vi "value_to_color.vi"(0 "Tab Control":enum32{"Page 1", "Page 2"}(tab)) -> ()   [LabVIEW 2019]
panel:
  in  "Rang":u16(ring) items=["10^-2", "10^-1", "10^0", "10^1", "10^2", "10^3", "10^4", "10^5", "10^6", "10^7", "10^8", "10^9"]
  in  "4B":bool
  in  "1B":bool
  in  "?":bool
  in  "Decimal value":dbl min=0.0 max=999.0 step=1.0
  in  "Thermal coefficient":u16(ring) items=["200"=200, "100"=100, "50"=50, "15"=15, "25"=25, "10"=10, "5"=5, "1"=1]
  in  "Precision":u16(ring) items=["20 %", "10 %", "5 %", "1 %", "2 %", "0,5 %", "0,25 %", "0,10 %", "0,05 %"]
  in  "6B":bool
  in  "5B":bool
  out "?":string
  in  "ok":bool
  out "L1":bool
  out "L4":bool
  out "L5":bool
  out "L6":bool
  out "L2":bool
  out "L3":bool
  # "Value                                                 Color"
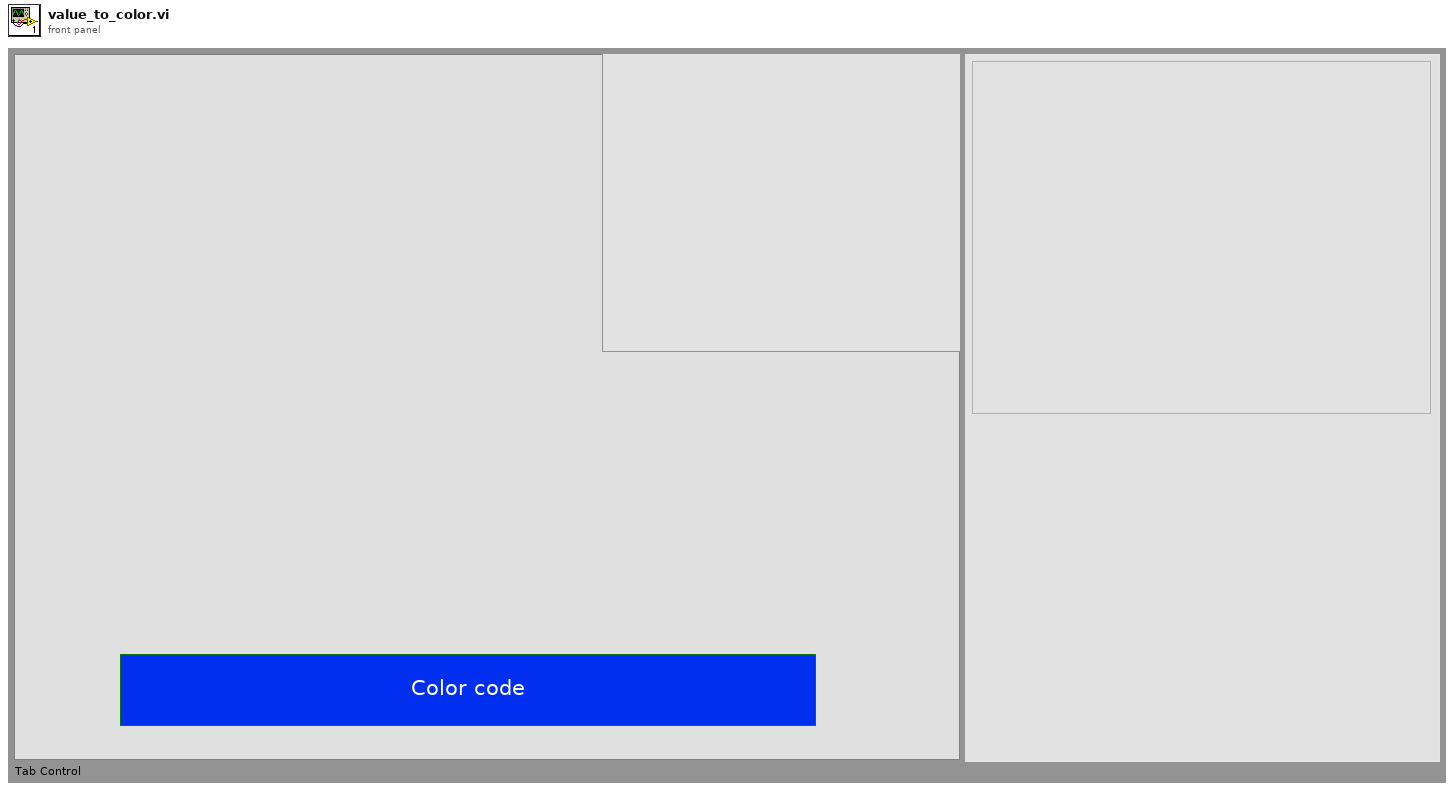
[diagram p1: front panel]
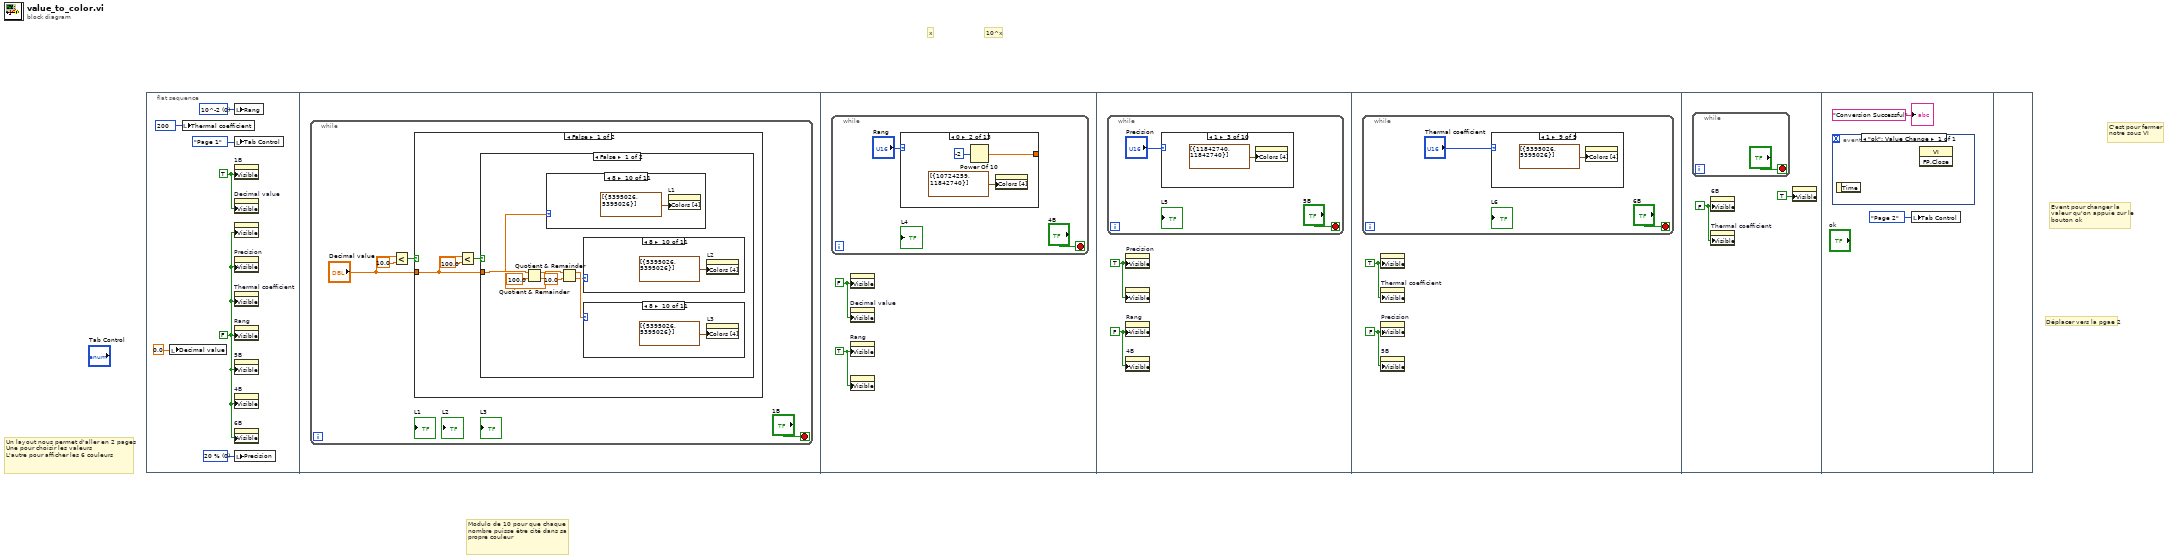
[diagram p0: block diagram]
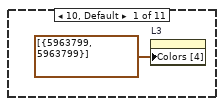
[diagram p2: hidden frame]
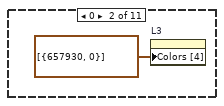
[diagram p3: hidden frame]
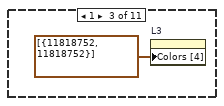
[diagram p4: hidden frame]
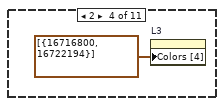
[diagram p5: hidden frame]
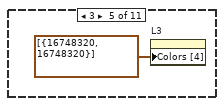
[diagram p6: hidden frame]
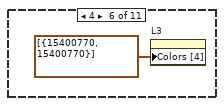
[diagram p7: hidden frame]
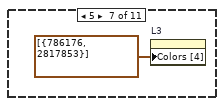
[diagram p8: hidden frame]
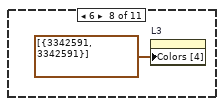
[diagram p9: hidden frame]
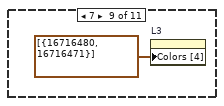
[diagram p10: hidden frame]
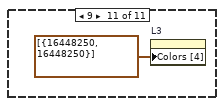
[diagram p11: hidden frame]
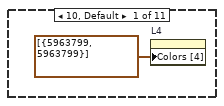
[diagram p12: hidden frame]
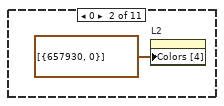
[diagram p13: hidden frame]
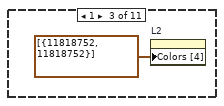
[diagram p14: hidden frame]
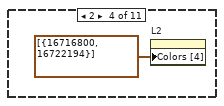
[diagram p15: hidden frame]
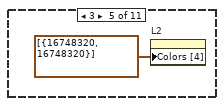
[diagram p16: hidden frame]
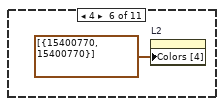
[diagram p17: hidden frame]
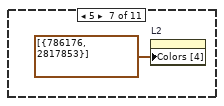
[diagram p18: hidden frame]
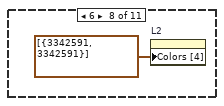
[diagram p19: hidden frame]
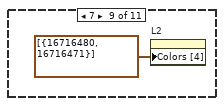
[diagram p20: hidden frame]
diagram:
  # "Déplacer vers la pgae 2"
  # "C'est pour fermer notre sous VI"
  # "Event pour changer la valeur qu'on appuie sur le bouton ok"
  # "x"
  # "10^x"
  # "Modulo de 10 pour que chaque nombre puisse être cité dans sa propre couleur"
  # "Un layout nous permet d'aller en 2 pages\nUne pour choisir les valeurs\nL'autre pour afficher les 6 couleurs"
  n1 = flat-sequence {
    frame #0 {
      w1 = u16 0 items=["20 %", "10 %", "5 %", "1 %", "2 %", "0,5 %", "0,25 %", "0,10 %", "0,05 %"] ("Precision")
      w2 = u16 0 items=["10^-2", "10^-1", "10^0", "10^1", "10^2", "10^3", "10^4", "10^5", "10^6", "10^7", "10^8", "10^9"] ("Rang")
      w3 = u16 200 items=["200"=200, "100"=100, "50"=50, "15"=15, "25"=25, "10"=10, "5"=5, "1"=1] ("Thermal coefficient")
      w7 = TRUE
      w5 = FALSE
      n2 = local write "Decimal value"(0.0 ("Decimal value")) -> ()
      n3 = local write "Thermal coefficient"(w3) -> ()
      n4 = local write "Rang"(w2) -> ()
      n5 = local write "Tab Control"(enum32{"Page 1", "Page 2"}."Page 1" ("Tab Control")) -> ()
      n6 = property on="1B" class="Bool"("Visible"=w7) -> ()  [unwired: 2 in, 2 out]
      n7 = property on="Decimal value" class="DigNum (strict)"("Visible"=w7) -> ()  [unwired: 2 in, 2 out]
      n8 = property class="Bool"("Visible"=w5) -> ()  [unwired: 2 in, 2 out]
      n9 = property on="Precision" class="Ring (strict)"("Visible"=w5) -> ()  [unwired: 2 in, 2 out]
      n10 = property on="Thermal coefficient" class="Ring (strict)"("Visible"=w5) -> ()  [unwired: 2 in, 2 out]
      n11 = property on="Rang" class="Ring (strict)"("Visible"=w5) -> ()  [unwired: 2 in, 2 out]
      n12 = property on="5B" class="Bool"("Visible"=w5) -> ()  [unwired: 2 in, 2 out]
      n13 = property on="4B" class="Bool"("Visible"=w5) -> ()  [unwired: 2 in, 2 out]
      n14 = property on="6B" class="Bool"("Visible"=w5) -> ()  [unwired: 2 in, 2 out]
      n15 = local write "Precision"(w1) -> ()
    }
    frame #1 {
      n16 = while {
        stop <- "1B" stop-if-true
        n17 = Less?(x="Decimal value", y=10.0) -> (x < y?=w8:bool)
        n18 = case shown="False" w8 {
          tunnel: "Decimal value" -> [w12 w84]
          frame False {
            n19 = Less?(x=w12, y=100.0) -> (x < y?=w13:bool)
            n20 = case shown="False" w13 {
              tunnel: w12 -> [w20 w58]
              frame False {
                n21 = Quotient & Remainder(x=w20, y=100.0) -> (x-y*floor(x/y)=w18:dbl, floor(x/y)=w19:dbl)
                n22 = case shown="8" w19 {
                  frame 10, Default {
                    n23 = property on="L1" class="Bool (strict)"("Colors [4]"=cluster{u32, u32}[] [{5963799, 5963799}]) -> ()  [unwired: 2 in, 2 out]
                  }
                  frame 0 {
                    n24 = property on="L1" class="Bool (strict)"("Colors [4]"=cluster{u32, u32}[] [{657930, 0}]) -> ()  [unwired: 2 in, 2 out]
                  }
                  frame 1 {
                    n25 = property on="L1" class="Bool (strict)"("Colors [4]"=cluster{u32, u32}[] [{11818752, 11818752}]) -> ()  [unwired: 2 in, 2 out]
                  }
                  frame 2 {
                    n26 = property on="L1" class="Bool (strict)"("Colors [4]"=cluster{u32, u32}[] [{16716800, 16722194}]) -> ()  [unwired: 2 in, 2 out]
                  }
                  frame 3 {
                    n27 = property on="L1" class="Bool (strict)"("Colors [4]"=cluster{u32, u32}[] [{16748320, 16748320}]) -> ()  [unwired: 2 in, 2 out]
                  }
                  frame 4 {
                    n28 = property on="L1" class="Bool (strict)"("Colors [4]"=cluster{u32, u32}[] [{15400770, 15400770}]) -> ()  [unwired: 2 in, 2 out]
                  }
                  frame 5 {
                    n29 = property on="L1" class="Bool (strict)"("Colors [4]"=cluster{u32, u32}[] [{786176, 2817853}]) -> ()  [unwired: 2 in, 2 out]
                  }
                  frame 6 {
                    n30 = property on="L1" class="Bool (strict)"("Colors [4]"=cluster{u32, u32}[] [{3342591, 3342591}]) -> ()  [unwired: 2 in, 2 out]
                  }
                  frame 7 {
                    n31 = property on="L1" class="Bool (strict)"("Colors [4]"=cluster{u32, u32}[] [{16716480, 16716471}]) -> ()  [unwired: 2 in, 2 out]
                  }
                  frame 8 {
                    n32 = property on="L1" class="Bool (strict)"("Colors [4]"=cluster{u32, u32}[] [{5395026, 5395026}]) -> ()  [unwired: 2 in, 2 out]
                  }
                  frame 9 {
                    n33 = property on="L1" class="Bool (strict)"("Colors [4]"=cluster{u32, u32}[] [{16448250, 16448250}]) -> ()  [unwired: 2 in, 2 out]
                  }
                }
                n34 = Quotient & Remainder(x=w18, y=10.0) -> (x-y*floor(x/y)=w16:dbl, floor(x/y)=w15:dbl)
                n35 = case shown="8" w15 {
                  frame 10, Default {
                    n36 = property on="L4" class="Bool (strict)"("Colors [4]"=cluster{u32, u32}[] [{5963799, 5963799}]) -> ()  [unwired: 2 in, 2 out]
                  }
                  frame 0 {
                    n37 = property on="L2" class="Bool (strict)"("Colors [4]"=cluster{u32, u32}[] [{657930, 0}]) -> ()  [unwired: 2 in, 2 out]
                  }
                  frame 1 {
                    n38 = property on="L2" class="Bool (strict)"("Colors [4]"=cluster{u32, u32}[] [{11818752, 11818752}]) -> ()  [unwired: 2 in, 2 out]
                  }
                  frame 2 {
                    n39 = property on="L2" class="Bool (strict)"("Colors [4]"=cluster{u32, u32}[] [{16716800, 16722194}]) -> ()  [unwired: 2 in, 2 out]
                  }
                  frame 3 {
                    n40 = property on="L2" class="Bool (strict)"("Colors [4]"=cluster{u32, u32}[] [{16748320, 16748320}]) -> ()  [unwired: 2 in, 2 out]
                  }
                  frame 4 {
                    n41 = property on="L2" class="Bool (strict)"("Colors [4]"=cluster{u32, u32}[] [{15400770, 15400770}]) -> ()  [unwired: 2 in, 2 out]
                  }
                  frame 5 {
                    n42 = property on="L2" class="Bool (strict)"("Colors [4]"=cluster{u32, u32}[] [{786176, 2817853}]) -> ()  [unwired: 2 in, 2 out]
                  }
                  frame 6 {
                    n43 = property on="L2" class="Bool (strict)"("Colors [4]"=cluster{u32, u32}[] [{3342591, 3342591}]) -> ()  [unwired: 2 in, 2 out]
                  }
                  frame 7 {
                    n44 = property on="L2" class="Bool (strict)"("Colors [4]"=cluster{u32, u32}[] [{16716480, 16716471}]) -> ()  [unwired: 2 in, 2 out]
                  }
                  frame 8 {
                    n45 = property on="L2" class="Bool (strict)"("Colors [4]"=cluster{u32, u32}[] [{5395026, 5395026}]) -> ()  [unwired: 2 in, 2 out]
                  }
                  frame 9 {
                    n46 = property on="L2" class="Bool (strict)"("Colors [4]"=cluster{u32, u32}[] [{16448250, 16448250}]) -> ()  [unwired: 2 in, 2 out]
                  }
                }
                n47 = case shown="8" w16 {
                  frame 10, Default {
                    n48 = property on="L3" class="Bool (strict)"("Colors [4]"=cluster{u32, u32}[] [{5963799, 5963799}]) -> ()  [unwired: 2 in, 2 out]
                  }
                  frame 0 {
                    n49 = property on="L3" class="Bool (strict)"("Colors [4]"=cluster{u32, u32}[] [{657930, 0}]) -> ()  [unwired: 2 in, 2 out]
                  }
                  frame 1 {
                    n50 = property on="L3" class="Bool (strict)"("Colors [4]"=cluster{u32, u32}[] [{11818752, 11818752}]) -> ()  [unwired: 2 in, 2 out]
                  }
                  frame 2 {
                    n51 = property on="L3" class="Bool (strict)"("Colors [4]"=cluster{u32, u32}[] [{16716800, 16722194}]) -> ()  [unwired: 2 in, 2 out]
                  }
                  frame 3 {
                    n52 = property on="L3" class="Bool (strict)"("Colors [4]"=cluster{u32, u32}[] [{16748320, 16748320}]) -> ()  [unwired: 2 in, 2 out]
                  }
                  frame 4 {
                    n53 = property on="L3" class="Bool (strict)"("Colors [4]"=cluster{u32, u32}[] [{15400770, 15400770}]) -> ()  [unwired: 2 in, 2 out]
                  }
                  frame 5 {
                    n54 = property on="L3" class="Bool (strict)"("Colors [4]"=cluster{u32, u32}[] [{786176, 2817853}]) -> ()  [unwired: 2 in, 2 out]
                  }
                  frame 6 {
                    n55 = property on="L3" class="Bool (strict)"("Colors [4]"=cluster{u32, u32}[] [{3342591, 3342591}]) -> ()  [unwired: 2 in, 2 out]
                  }
                  frame 7 {
                    n56 = property on="L3" class="Bool (strict)"("Colors [4]"=cluster{u32, u32}[] [{16716480, 16716471}]) -> ()  [unwired: 2 in, 2 out]
                  }
                  frame 8 {
                    n57 = property on="L3" class="Bool (strict)"("Colors [4]"=cluster{u32, u32}[] [{5395026, 5395026}]) -> ()  [unwired: 2 in, 2 out]
                  }
                  frame 9 {
                    n58 = property on="L3" class="Bool (strict)"("Colors [4]"=cluster{u32, u32}[] [{16448250, 16448250}]) -> ()  [unwired: 2 in, 2 out]
                  }
                }
              }
              frame True {
                n59 = Quotient & Remainder(x=w58, y=10.0) -> (x-y*floor(x/y)=w56:dbl, floor(x/y)=w55:dbl)
                n60 = case shown="8" w56 {
                  frame 10, Default {
                    (unwired) nan
                    n61 = property on="L3" class="Bool (strict)"("Colors [4]"=cluster{u32, u32}[] [{5963799, 5963799}]) -> ()  [unwired: 2 in, 2 out]
                  }
                  frame 0 {
                    (unwired) 0
                    n62 = property on="L3" class="Bool (strict)"("Colors [4]"=cluster{u32, u32}[] [{657930, 0}]) -> ()  [unwired: 2 in, 2 out]
                  }
                  frame 1 {
                    (unwired) 1
                    n63 = property on="L3" class="Bool (strict)"("Colors [4]"=cluster{u32, u32}[] [{11818752, 11818752}]) -> ()  [unwired: 2 in, 2 out]
                  }
                  frame 2 {
                    (unwired) 2
                    n64 = property on="L3" class="Bool (strict)"("Colors [4]"=cluster{u32, u32}[] [{16716800, 16722194}]) -> ()  [unwired: 2 in, 2 out]
                  }
                  frame 3 {
                    n65 = property on="L3" class="Bool (strict)"("Colors [4]"=cluster{u32, u32}[] [{16748320, 16748320}]) -> ()  [unwired: 2 in, 2 out]
                  }
                  frame 4 {
                    n66 = property on="L3" class="Bool (strict)"("Colors [4]"=cluster{u32, u32}[] [{15400770, 15400770}]) -> ()  [unwired: 2 in, 2 out]
                  }
                  frame 5 {
                    n67 = property on="L3" class="Bool (strict)"("Colors [4]"=cluster{u32, u32}[] [{786176, 2817853}]) -> ()  [unwired: 2 in, 2 out]
                  }
                  frame 6 {
                    n68 = property on="L3" class="Bool (strict)"("Colors [4]"=cluster{u32, u32}[] [{3342591, 3342591}]) -> ()  [unwired: 2 in, 2 out]
                  }
                  frame 7 {
                    n69 = property on="L3" class="Bool (strict)"("Colors [4]"=cluster{u32, u32}[] [{16716480, 16716471}]) -> ()  [unwired: 2 in, 2 out]
                  }
                  frame 8 {
                    n70 = property on="L3" class="Bool (strict)"("Colors [4]"=cluster{u32, u32}[] [{5395026, 5395026}]) -> ()  [unwired: 2 in, 2 out]
                  }
                  frame 9 {
                    n71 = property on="L3" class="Bool (strict)"("Colors [4]"=cluster{u32, u32}[] [{16448250, 16448250}]) -> ()  [unwired: 2 in, 2 out]
                  }
                }
                n72 = case shown="8" w55 {
                  frame 10, Default {
                    n73 = property on="L2" class="Bool (strict)"("Colors [4]"=cluster{u32, u32}[] [{5963799, 5963799}]) -> ()  [unwired: 2 in, 2 out]
                  }
                  frame 0 {
                    n74 = property on="L2" class="Bool (strict)"("Colors [4]"=cluster{u32, u32}[] [{657930, 0}]) -> ()  [unwired: 2 in, 2 out]
                  }
                  frame 1 {
                    n75 = property on="L2" class="Bool (strict)"("Colors [4]"=cluster{u32, u32}[] [{11818752, 11818752}]) -> ()  [unwired: 2 in, 2 out]
                  }
                  frame 2 {
                    n76 = property on="L2" class="Bool (strict)"("Colors [4]"=cluster{u32, u32}[] [{16716800, 16722194}]) -> ()  [unwired: 2 in, 2 out]
                  }
                  frame 3 {
                    n77 = property on="L2" class="Bool (strict)"("Colors [4]"=cluster{u32, u32}[] [{16748320, 16748320}]) -> ()  [unwired: 2 in, 2 out]
                  }
                  frame 4 {
                    n78 = property on="L2" class="Bool (strict)"("Colors [4]"=cluster{u32, u32}[] [{15400770, 15400770}]) -> ()  [unwired: 2 in, 2 out]
                  }
                  frame 5 {
                    n79 = property on="L2" class="Bool (strict)"("Colors [4]"=cluster{u32, u32}[] [{786176, 2817853}]) -> ()  [unwired: 2 in, 2 out]
                  }
                  frame 6 {
                    n80 = property on="L2" class="Bool (strict)"("Colors [4]"=cluster{u32, u32}[] [{3342591, 3342591}]) -> ()  [unwired: 2 in, 2 out]
                  }
                  frame 7 {
                    n81 = property on="L2" class="Bool (strict)"("Colors [4]"=cluster{u32, u32}[] [{16716480, 16716471}]) -> ()  [unwired: 2 in, 2 out]
                  }
                  frame 8 {
                    n82 = property on="L2" class="Bool (strict)"("Colors [4]"=cluster{u32, u32}[] [{5395026, 5395026}]) -> ()  [unwired: 2 in, 2 out]
                  }
                  frame 9 {
                    n83 = property on="L2" class="Bool (strict)"("Colors [4]"=cluster{u32, u32}[] [{16448250, 16448250}]) -> ()  [unwired: 2 in, 2 out]
                  }
                }
                n84 = property on="L1" class="Bool (strict)"("Colors [4]"=cluster{u32, u32}[] [{0, 0}]) -> ()  [unwired: 2 in, 2 out]
              }
            }
          }
          frame True {
            n85 = case shown="8" w84 {
              frame 10, Default {
                n86 = property on="L3" class="Bool (strict)"("Colors [4]"=cluster{u32, u32}[] [{5963799, 5963799}]) -> ()  [unwired: 2 in, 2 out]
              }
              frame 0 {
                n87 = property on="L3" class="Bool (strict)"("Colors [4]"=cluster{u32, u32}[] [{657930, 0}]) -> ()  [unwired: 2 in, 2 out]
              }
              frame 1 {
                n88 = property on="L3" class="Bool (strict)"("Colors [4]"=cluster{u32, u32}[] [{11818752, 11818752}]) -> ()  [unwired: 2 in, 2 out]
              }
              frame 2 {
                n89 = property on="L3" class="Bool (strict)"("Colors [4]"=cluster{u32, u32}[] [{16716800, 16722194}]) -> ()  [unwired: 2 in, 2 out]
              }
              frame 3 {
                n90 = property on="L3" class="Bool (strict)"("Colors [4]"=cluster{u32, u32}[] [{16748320, 16748320}]) -> ()  [unwired: 2 in, 2 out]
              }
              frame 4 {
                n91 = property on="L3" class="Bool (strict)"("Colors [4]"=cluster{u32, u32}[] [{15400770, 15400770}]) -> ()  [unwired: 2 in, 2 out]
              }
              frame 5 {
                n92 = property on="L3" class="Bool (strict)"("Colors [4]"=cluster{u32, u32}[] [{786176, 2817853}]) -> ()  [unwired: 2 in, 2 out]
              }
              frame 6 {
                n93 = property on="L3" class="Bool (strict)"("Colors [4]"=cluster{u32, u32}[] [{3342591, 3342591}]) -> ()  [unwired: 2 in, 2 out]
              }
              frame 7 {
                n94 = property on="L3" class="Bool (strict)"("Colors [4]"=cluster{u32, u32}[] [{16716480, 16716471}]) -> ()  [unwired: 2 in, 2 out]
              }
              frame 8 {
                n95 = property on="L3" class="Bool (strict)"("Colors [4]"=cluster{u32, u32}[] [{5395026, 5395026}]) -> ()  [unwired: 2 in, 2 out]
              }
              frame 9 {
                n96 = property on="L3" class="Bool (strict)"("Colors [4]"=cluster{u32, u32}[] [{16448250, 16448250}]) -> ()  [unwired: 2 in, 2 out]
              }
            }
            n97 = property on="L1" class="Bool (strict)"("Colors [4]"=cluster{u32, u32}[] [{0, 65793}]) -> ()  [unwired: 2 in, 2 out]
            n98 = property on="L2" class="Bool (strict)"("Colors [4]"=cluster{u32, u32}[] [{0, 0}]) -> ()  [unwired: 2 in, 2 out]
          }
        }
      }
    }
    frame #2 {
      w97 = TRUE
      w96 = FALSE
      n99 = while {
        stop <- "4B" stop-if-true
        n100 = case shown="0" "Rang" {
          tunnel: [1.0 w102 w105 w108 w111 w114 w117 w120 w123 w126 w129 w132 w135] -> _
          frame 12, Default {
            n101 = property on="L4" class="Bool (strict)"("Colors [4]"=cluster{u32, u32}[] [{5963799, 5963799}]) -> ()  [unwired: 2 in, 2 out]
          }
          frame 0 {
            n102 = Power Of 10(x=-2) -> (10^x=w102:dbl)
            n103 = property on="L4" class="Bool (strict)"("Colors [4]"=cluster{u32, u32}[] [{10724259, 11842740}]) -> ()  [unwired: 2 in, 2 out]
          }
          frame 1 {
            n104 = Power Of 10(x=-1) -> (10^x=w105:dbl)
            n105 = property on="L4" class="Bool (strict)"("Colors [4]"=cluster{u32, u32}[] [{16763714, 16756736}]) -> ()  [unwired: 2 in, 2 out]
          }
          frame 2 {
            n106 = property on="L4" class="Bool (strict)"("Colors [4]"=cluster{u32, u32}[] [{0, 263172}]) -> ()  [unwired: 2 in, 2 out]
            n107 = Power Of 10(x=0) -> (10^x=w108:dbl)
          }
          frame 3 {
            n108 = property on="L4" class="Bool (strict)"("Colors [4]"=cluster{u32, u32}[] [{13128704, 13128704}]) -> ()  [unwired: 2 in, 2 out]
            n109 = Power Of 10(x=1) -> (10^x=w111:dbl)
          }
          frame 4 {
            n110 = property on="L4" class="Bool (strict)"("Colors [4]"=cluster{u32, u32}[] [{16716800, 16722194}]) -> ()  [unwired: 2 in, 2 out]
            n111 = Power Of 10(x=2) -> (10^x=w114:dbl)
          }
          frame 5 {
            n112 = property on="L4" class="Bool (strict)"("Colors [4]"=cluster{u32, u32}[] [{16748320, 16748320}]) -> ()  [unwired: 2 in, 2 out]
            n113 = Power Of 10(x=3) -> (10^x=w117:dbl)
          }
          frame 6 {
            n114 = property on="L4" class="Bool (strict)"("Colors [4]"=cluster{u32, u32}[] [{15400770, 15400770}]) -> ()  [unwired: 2 in, 2 out]
            n115 = Power Of 10(x=4) -> (10^x=w120:dbl)
          }
          frame 7 {
            n116 = property on="L4" class="Bool (strict)"("Colors [4]"=cluster{u32, u32}[] [{786176, 2817853}]) -> ()  [unwired: 2 in, 2 out]
            n117 = Power Of 10(x=5) -> (10^x=w123:dbl)
          }
          frame 8 {
            n118 = property on="L4" class="Bool (strict)"("Colors [4]"=cluster{u32, u32}[] [{3342591, 3342591}]) -> ()  [unwired: 2 in, 2 out]
            n119 = Power Of 10(x=6) -> (10^x=w126:dbl)
          }
          frame 9 {
            n120 = property on="L4" class="Bool (strict)"("Colors [4]"=cluster{u32, u32}[] [{16716480, 16716471}]) -> ()  [unwired: 2 in, 2 out]
            n121 = Power Of 10(x=7) -> (10^x=w129:dbl)
          }
          frame 10 {
            n122 = property on="L4" class="Bool (strict)"("Colors [4]"=cluster{u32, u32}[] [{5395026, 5395026}]) -> ()  [unwired: 2 in, 2 out]
            n123 = Power Of 10(x=8) -> (10^x=w132:dbl)
          }
          frame 11 {
            n124 = property on="L4" class="Bool (strict)"("Colors [4]"=cluster{u32, u32}[] [{16448250, 16448250}]) -> ()  [unwired: 2 in, 2 out]
            n125 = Power Of 10(x=9) -> (10^x=w135:dbl)
          }
        }
      }
      n126 = property on="1B" class="Bool"("Visible"=w96) -> ()  [unwired: 2 in, 2 out]
      n127 = property on="Decimal value" class="DigNum (strict)"("Visible"=w96) -> ()  [unwired: 2 in, 2 out]
      n128 = property on="Rang" class="Ring (strict)"("Visible"=w97) -> ()  [unwired: 2 in, 2 out]
      n129 = property on="4B" class="Bool"("Visible"=w97) -> ()  [unwired: 2 in, 2 out]
    }
    frame #3 {
      w138 = TRUE
      w139 = FALSE
      n130 = while {
        stop <- "5B" stop-if-true
        n131 = case shown="1" "Precision" {
          frame 9, Default {
            n132 = property on="L5" class="Bool (strict)"("Colors [4]"=cluster{u32, u32}[] [{5963799, 5963799}]) -> ()  [unwired: 2 in, 2 out]
          }
          frame 0 {
            n133 = property on="L5" class="Bool (strict)"("Colors [4]"=cluster{u32, u32}[] [{16448250, 16448250}]) -> ()  [unwired: 2 in, 2 out]
          }
          frame 1 {
            n134 = property on="L5" class="Bool (strict)"("Colors [4]"=cluster{u32, u32}[] [{11842740, 11842740}]) -> ()  [unwired: 2 in, 2 out]
          }
          frame 2 {
            n135 = property on="L5" class="Bool (strict)"("Colors [4]"=cluster{u32, u32}[] [{16366338, 16366338}]) -> ()  [unwired: 2 in, 2 out]
          }
          frame 3 {
            n136 = property on="L5" class="Bool (strict)"("Colors [4]"=cluster{u32, u32}[] [{13128704, 13128704}]) -> ()  [unwired: 2 in, 2 out]
          }
          frame 4 {
            n137 = property on="L5" class="Bool (strict)"("Colors [4]"=cluster{u32, u32}[] [{16716800, 16722194}]) -> ()  [unwired: 2 in, 2 out]
          }
          frame 5 {
            n138 = property on="L5" class="Bool (strict)"("Colors [4]"=cluster{u32, u32}[] [{3079978, 3079978}]) -> ()  [unwired: 2 in, 2 out]
          }
          frame 6 {
            n139 = property on="L5" class="Bool (strict)"("Colors [4]"=cluster{u32, u32}[] [{458911, 327880}]) -> ()  [unwired: 2 in, 2 out]
          }
          frame 7 {
            n140 = property on="L5" class="Bool (strict)"("Colors [4]"=cluster{u32, u32}[] [{16711894, 15663313}]) -> ()  [unwired: 2 in, 2 out]
          }
          frame 8 {
            n141 = property on="L5" class="Bool (strict)"("Colors [4]"=cluster{u32, u32}[] [{5395026, 5395026}]) -> ()  [unwired: 2 in, 2 out]
          }
        }
      }
      n142 = property on="Precision" class="Ring (strict)"("Visible"=w138) -> ()  [unwired: 2 in, 2 out]
      n143 = property on="5B" class="Bool"("Visible"=w138) -> ()  [unwired: 2 in, 2 out]
      n144 = property on="Rang" class="Ring (strict)"("Visible"=w139) -> ()  [unwired: 2 in, 2 out]
      n145 = property on="4B" class="Bool"("Visible"=w139) -> ()  [unwired: 2 in, 2 out]
    }
    frame #4 {
      w153 = TRUE
      w152 = FALSE
      n146 = while {
        stop <- "6B" stop-if-true
        n147 = case shown="1" "Thermal coefficient" {
          frame 8, Default {
            n148 = property on="L6" class="Bool (strict)"("Colors [4]"=cluster{u32, u32}[] [{5963799, 5963799}]) -> ()  [unwired: 2 in, 2 out]
          }
          frame 200 {
            n149 = property on="L6" class="Bool (strict)"("Colors [4]"=cluster{u32, u32}[] [{657930, 0}]) -> ()  [unwired: 2 in, 2 out]
          }
          frame 100 {
            n150 = property on="L6" class="Bool (strict)"("Colors [4]"=cluster{u32, u32}[] [{11818752, 11818752}]) -> ()  [unwired: 2 in, 2 out]
          }
          frame 50 {
            n151 = property on="L6" class="Bool (strict)"("Colors [4]"=cluster{u32, u32}[] [{16716800, 16722194}]) -> ()  [unwired: 2 in, 2 out]
          }
          frame 15 {
            n152 = property on="L6" class="Bool (strict)"("Colors [4]"=cluster{u32, u32}[] [{16748320, 16748320}]) -> ()  [unwired: 2 in, 2 out]
          }
          frame 25 {
            n153 = property on="L6" class="Bool (strict)"("Colors [4]"=cluster{u32, u32}[] [{15400770, 15400770}]) -> ()  [unwired: 2 in, 2 out]
          }
          frame 10 {
            n154 = property on="L6" class="Bool (strict)"("Colors [4]"=cluster{u32, u32}[] [{393471, 6380031}]) -> ()  [unwired: 2 in, 2 out]
          }
          frame 5 {
            n155 = property on="L6" class="Bool (strict)"("Colors [4]"=cluster{u32, u32}[] [{16716480, 16711885}]) -> ()  [unwired: 2 in, 2 out]
          }
          frame 1 {
            n156 = property on="L6" class="Bool (strict)"("Colors [4]"=cluster{u32, u32}[] [{5395026, 5395026}]) -> ()  [unwired: 2 in, 2 out]
          }
        }
      }
      n157 = property on="6B" class="Bool"("Visible"=w153) -> ()  [unwired: 2 in, 2 out]
      n158 = property on="Thermal coefficient" class="Ring (strict)"("Visible"=w153) -> ()  [unwired: 2 in, 2 out]
      n159 = property on="Precision" class="Ring (strict)"("Visible"=w152) -> ()  [unwired: 2 in, 2 out]
      n160 = property on="5B" class="Bool"("Visible"=w152) -> ()  [unwired: 2 in, 2 out]
    }
    frame #5 {
      w166 = FALSE
      n161 = while {
        stop <- "?" stop-if-true
      }
      n162 = property on="6B" class="Bool"("Visible"=w166) -> ()  [unwired: 2 in, 2 out]
      n163 = property on="Thermal coefficient" class="Ring (strict)"("Visible"=w166) -> ()  [unwired: 2 in, 2 out]
      n164 = property class="Bool"("Visible"=TRUE) -> ()  [unwired: 2 in, 2 out]
    }
    frame #6 {
      n165 = event shown="[0] \"ok\": Value Change" {
        selector: _ -> [_]
        dyn-events: _ -> [_]
        timeout: _ -> [_]
        event "ok": Value Change {
          n166 = event-data() -> ()  [unwired: 1 in, 1 out]
          n167 = invoke class="VI" method="FP.Close"() -> ()  [unwired: 3 in, 3 out]
        }
      }
      n168 = local write "Tab Control"(enum32{"Page 1", "Page 2"}."Page 2" ("Tab Control")) -> ()
      "?" <- "Conversion Successful" ("String")
    }
    frame #7 {
    }
  }
